vi "Insert Public API VIS.vi"(7 "Application in":refnum<vi>, 10 "Tree Map in":T1, 11 "Library In":refnum<class "Library.lvclass">) -> (2 "Tree Map Out":T1, 3 "Library Out":refnum<class "Library.lvclass">)   [LabVIEW 2019, in "Panther Dashboard.lvlib"]
uses:
  Panther Dashboard.lvlib
  <vilib>/National Instruments/Tree Map/Tree Map Data.ctl
  Map Attribute--enum.ctl
  <vilib>/National Instruments/Tree Map/Tree Map.lvlib
  Class/VI/VI.lvclass
  Class/Library/Library.lvclass
panel:
  in  "Root path":string
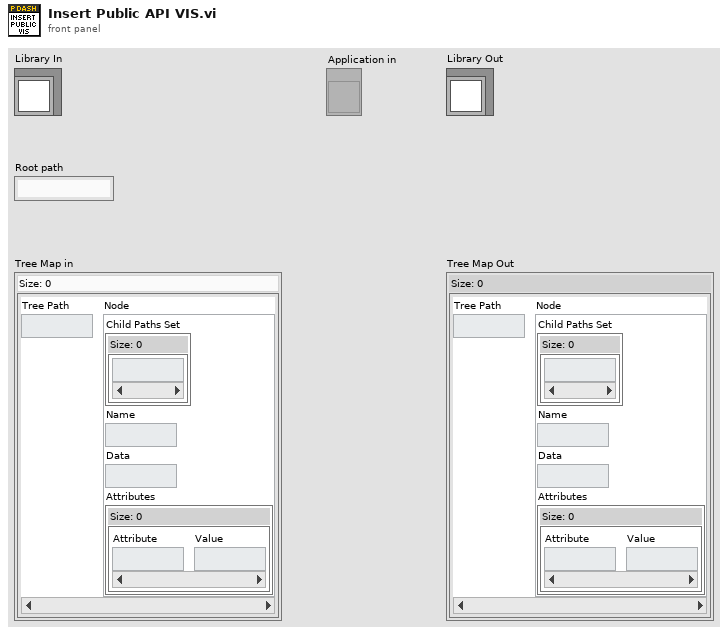
[diagram p1: front panel]
types:
  T1 = typedef "Tree Map.lvlib/Tree Map Data.ctl" = map{string, cluster{"Child Paths Set":set{string}, "Name":string, "Data":string, "Attributes":map{string, string}}}
  T2 = typedef "Panther Dashboard.lvlib/Map Attribute--enum.ctl" = enum16{"Path", "ModuleType", "Module Description", "Dependency?", "Target"}
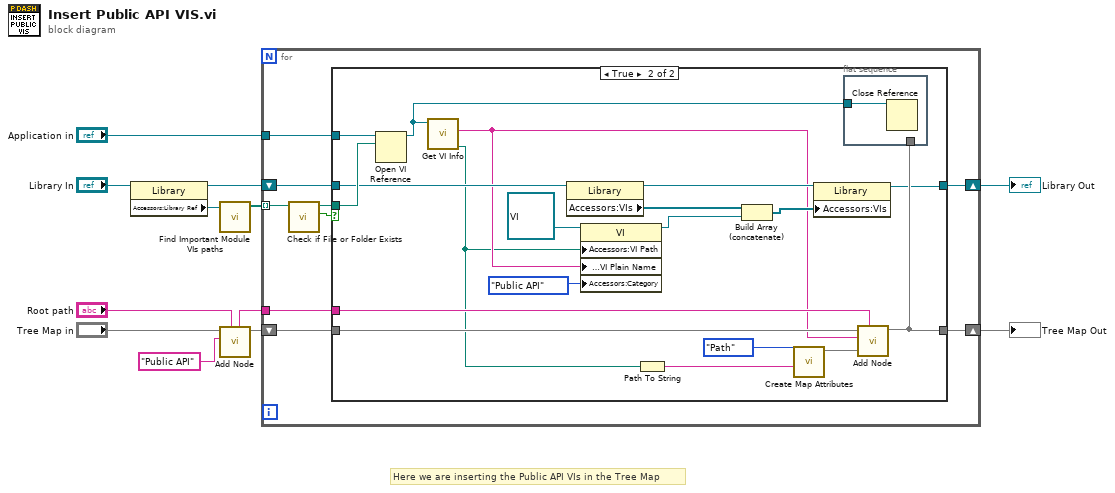
[diagram p0: block diagram]
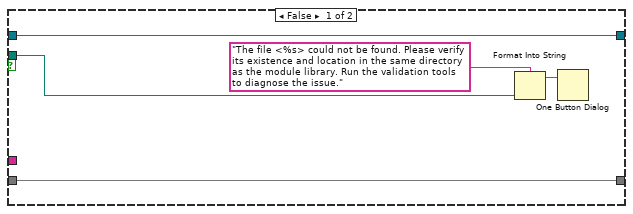
[diagram p2: hidden frame]
diagram:
  # "Here we are inserting the Public API VIs in the Tree Map"
  n1 = property class="Library"(reference="Library In") -> (reference out=w2:refnum<class "Library.lvclass">, "Accessors:Library Ref"=w3:refnum<vi>)  [unwired: 1 in, 1 out]
  n2 = call "Find Important Module VIs paths.vi"("Library in"=w3) -> ("Public API VIs Paths"=w11:path[])  [unwired: 10 in]
  n3 = call <vilib>:"Add Node.vi"("Parent Path"="Root path", "New Node Name"="Public API", "Tree Map In"="Tree Map in") -> ("Tree Map Out"=w7:T1, "New Node Path"=w5:string)  [unwired: 6 in, 1 out]
  n4 = for {
    tunnel: "Application in" -> [w21]
    tunnel: w11 -> [w17] mode=indexing
    shift-right: [w20] -> w10
    shift-left: w7 -> [w19]
    tunnel: w5 -> [w18]
    shift-right: [w13] -> w1
    shift-left: w2 -> [w14]
    n5 = call <vilib>:"Check if File or Folder Exists.vi"("path"=w17) -> ("file or folder exists?"=w16:bool, "dup path"=w15:path)  [unwired: 8 in, 1 out]
    n6 = case shown="True" w16 {
      tunnel: w21 -> [_ w45]
      tunnel: [w26 w37] -> w20
      tunnel: w19 -> [w26 w44]
      tunnel: w18 -> [_ w43]
      tunnel: w15 -> [w25 w42]
      tunnel: w14 -> [w22 w36]
      tunnel: [w22 w34] -> w13
      frame False {
        n7 = Format Into String(format string="The file <%s> could not be found. Please verify its existence and location in the same directory as the module library. Run the validation tools to diagnose the issue.", w25) -> (resulting string=w24:string)  [unwired: 2 in, 1 out]
        n8 = One Button Dialog(message=w24) -> ()  [unwired: 1 in, 1 out]
      }
      frame True {
        n9 = Open VI Reference(application reference (local)=w45, vi path=w42) -> (vi reference=w38:refnum<vi>)  [unwired: 4 in, 1 out]
        n10 = call "Get VI Info.vi"("VI in"=w38) -> ("VI Path"=w28:path, "Plain Name"=w29:string)  [unwired: 7 in, 2 out]
        n11 = property class="Library"(reference=w36) -> (reference out=w35:refnum<class "Library.lvclass">, "Accessors:VIs"=w33:refnum<class "VI.lvclass">[])  [unwired: 1 in, 1 out]
        n12 = property class="VI"(reference=refnum<class "VI.lvclass"> refnum ("array"), "Accessors:VI Path"=w28, "Accessors:VI Plain Name"=w29, "Accessors:Category"=enum16{"Public API", "Constant VI", "Error VI"}."Public API" ("Category")) -> (reference out=w30:refnum<class "VI.lvclass">)  [unwired: 1 in, 1 out]
        n13 = Path To String(path=w28) -> (string=w40:string)
        n14 = Build Array (concatenate)(w33, w30) -> (w32:refnum<class "VI.lvclass">[])
        n15 = call "Create Map Attributes.vi"("Attribute"=w40, "Map Attribute"=Map_Attribute--enum."Path") -> ("Root Attributes"=w39:map{string, string})  [unwired: 9 in]
        n16 = property class="Library"(reference=w35, "Accessors:VIs"=w32) -> (reference out=w34:refnum<class "Library.lvclass">)  [unwired: 1 in, 1 out]
        n17 = flat-sequence {
          tunnel: w38 -> [w46]
          tunnel: w37 -> [_]
          frame #0 {
            n18 = Close Reference(reference=w46) -> ()  [unwired: 1 in, 1 out]
          }
        }
        n19 = call <vilib>:"Add Node.vi"("Parent Path"=w43, "Attributes"=w39, "New Node Name"=w29, "Tree Map In"=w44) -> ("Tree Map Out"=w37:T1)  [unwired: 5 in, 2 out]
      }
    }
  }
  "Tree Map Out" <- w10
  "Library Out" <- w1
